vi "Data Log Refresh.vi"(8 "error in (no error)":errorcluster, 11 "Data Cluster":T1) -> (0 "error out":errorcluster)   [LabVIEW 2025]
uses:
  controls/LAB-IQ UI Data.ctl
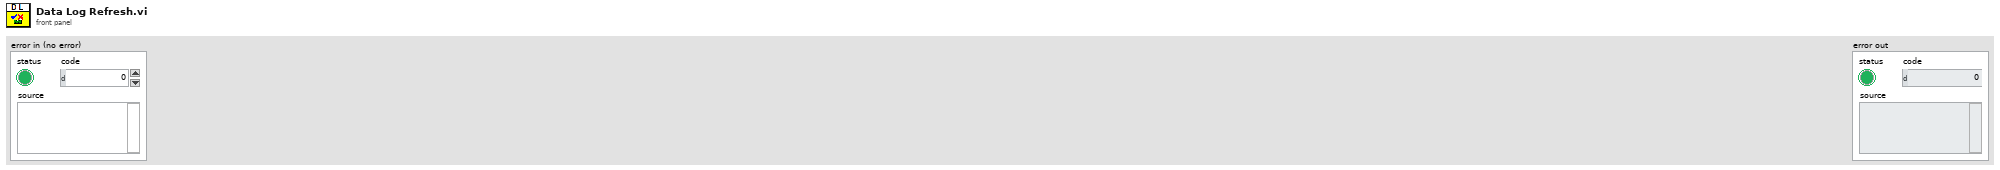
[diagram p1: front panel]
types:
  T1 = typedef "LAB-IQ UI Data.ctl" = cluster{"Main Home Screen":cluster{"GUI":refnum<vi>, "Platform Settings":refnum<vi>, "Configure":refnum<vi>, "Home":refnum<vi>, "EXIT":refnum<vi>, "service 2":refnum<vi>, "MainPage":refnum<vi>, "Analysis":refnum<vi>}, "Platform Settings":cluster{"mm/s  Surge":refnum<vi>, "Update Surge Speed":refnum<vi>, "Drive Error":refnum<vi>, "Disable Axis Jog Soft Limits":refnum<vi>, "mm/s  Sway":refnum<vi>, "Sway and Surge COM Status":refnum<vi>, "Heave COM Status":refnum<vi>, "Enable Platform":refnum<vi>, "Surge Forward Main":refnum<vi>, "Sway Right Main":refnum<vi>, "Sway Left Main":refnum<vi>, "Heave Down Main":refnum<vi>, "Heave Up main":refnum<vi>, "Update Sway Speed":refnum<vi>, "Update Heave Speed":refnum<vi>, "mm/s Heave":refnum<vi>, "mm/sec":refnum<vi>, "mm":refnum<vi>, "Surge Backward Main":refnum<vi>}, "Analysis Screen":cluster{"Analysis Home":refnum<vi>, "Surface Analysis":refnum<vi>, "Imaging":refnum<vi>, "Image Analysis":refnum<vi>, "Post Analysis":refnum<vi>}, "Config Screen":cluster{"Select Load Head":refnum<vi>, "Notes :":refnum<vi>, "FILE":refnum<vi>, "Sample ID :":refnum<vi>, "Operator ID :":refnum<vi>, "Operator Name :":refnum<vi>, "Auto":refnum<vi>}, "Motion Module":cluster{"zNL":refnum<vi>, "NL disp":refnum<vi>, "Rotary Tab":refnum<vi>, "Motion Direction:  3":refnum<vi>, "E.Velocity 2":refnum<vi>, "e.v/ssr 2":refnum<vi>, "Enter Fixed E.Velocity 2":refnum<vi>, "Enter Final SRR 2":refnum<vi>, "Enter initial SRR 2":refnum<vi>, "Enter Fixed SRR 2":refnum<vi>, "Enter the Final E.Velocity (m/s) 2":refnum<vi>, "Enter initial E.Velocity (m/s) 2":refnum<vi>, "Final Speed (RPM) 3":refnum<vi>, "Initial Speed (RPM) 2":refnum<vi>, "Enter the Final Velocity (m/s) 3":refnum<vi>, "Enter initial Velocity (m/s)  3":refnum<vi>, "Ramp Up 2":refnum<vi>, "TEST SELECTION":refnum<vi>, "SPEED SELECTION : ":refnum<vi>, "Angular Oscillation Set":refnum<vi>, "Traction":refnum<vi>, "Step Speed":refnum<vi>, "StepTable For Load-Speed":refnum<vi>, "StepTable For Speed":refnum<vi>, "Surge Forward MM":refnum<vi>, "Surge Backward MM":refnum<vi>, "M3 Image":refnum<vi>, "String 39":refnum<vi>, "Sway Left MM":refnum<vi>, "Sway Right MM":refnum<vi>, "Disable Axis Jog Soft Limits":refnum<vi>, "mm":refnum<vi>, "Heave Down MM":refnum<vi>, "Heave Up MM":refnum<vi>, "Wear Track Diameter (mm)":refnum<vi>, "Set WTD":refnum<vi>, "HomeScratch":refnum<vi>, "HomeRot":refnum<vi>, "PlaceModule":refnum<vi>, "Enter the Angle (Deg)":refnum<vi>, "Enter the Frequency (Hz)":refnum<vi>, "Motion Mode:":refnum<vi>, "LR Sway":refnum<vi>, "Rot Hor":refnum<vi>, "Scratch":refnum<vi>, "LR Cam":refnum<vi>, "MMBack":refnum<vi>, "MMNext":refnum<vi>, "Rot Ver":refnum<vi>, "Rotary Module Selection":refnum<vi>, "calculate rotary":refnum<vi>, "SPEED SELECTION : rotary":refnum<vi>, "Import 2":refnum<vi>, "Save 2":refnum<vi>, "File Path :  2":refnum<vi>, "String 45":refnum<vi>, "StepTable For Speed 3":refnum<vi>, "Enter the Speed(mm/sec)":refnum<vi>, "Enter the Speed(RPM)":refnum<vi>, "Enter Scratch Speed (mm/s):":refnum<vi>, "SwaySpeed Set":refnum<vi>, "Scartch Offset":refnum<vi>, "Motion type:":refnum<vi>, "HomeScratch 2":refnum<vi>, "Enter Scratch length (mm):":refnum<vi>, "Wear Track Diameter":refnum<vi>, "Rotary Speed Exced":refnum<vi>, "Scratch Mode":refnum<vi>, "No of Scratch":refnum<vi>}, "Environmental control":cluster{"Humidity  Status  3":refnum<vi>, "Low Temp  Status  2":refnum<vi>, "TK4 status 2":refnum<vi>, "Stage Temperature":refnum<vi>, "Sample Temperature":refnum<vi>, "Humidity (Amb)":refnum<vi>, "Clear List":refnum<vi>, "Add to list":refnum<vi>, "Wear":refnum<vi>, "Vibration":refnum<vi>, "Humidity (Chamber)":refnum<vi>, "Temperature (Chamber)":refnum<vi>, "ECR ":refnum<vi>, "Temperature (Amb)":refnum<vi>, "Microphone":refnum<vi>, "Acoustic Emission 3":refnum<vi>, "SNext":refnum<vi>, "APBack":refnum<vi>, "Enter the Temperature (°C):":refnum<vi>, "Enter the Stage \nTemperature (°C):":refnum<vi>, "Enter the Humidity (%Rh):":refnum<vi>, "Low Temp":refnum<vi>, "High Temp":refnum<vi>, "Humidity":refnum<vi>, "Sensors Picked":refnum<vi>}, "About Screen":cluster{"Password":refnum<vi>, "Home Service":refnum<vi>, "Advanced Setting":refnum<vi>, "About Tab":refnum<vi>, "ECR Port:":refnum<vi>, "Ramp Port:":refnum<vi>, "Installation/Replacement completed":refnum<vi>, "Loahead":refnum<vi>, "Heave and Surge COM Port:":refnum<vi>, "Sway COM Port:":refnum<vi>, "Temp Modbus:":refnum<vi>, "Humidity Port:":refnum<vi>, "Edit Gain Constants":refnum<vi>, "Save Gain Constants":refnum<vi>}, "Main Screen":cluster{"Main Screen Tab":refnum<vi>, "Angle and Frequency":refnum<vi>, "Stroke (mm)":refnum<vi>, "Angle (Deg)":refnum<vi>, "Main Speed Tab":refnum<vi>, "MTM MOTOR DISPLAY":refnum<vi>, "Disc Speed (m/sec)":refnum<vi>, "Ball Speed (m/sec)":refnum<vi>, "Disc Speed (RPM)":refnum<vi>, "Ball Speed (RPM)":refnum<vi>, "SPEED TAB":refnum<vi>, "Speed (m/sec)":refnum<vi>, "Set Speed (m/sec)":refnum<vi>, "Speed (RPM)":refnum<vi>, "Set Speed":refnum<vi>, "Time Tab":refnum<vi>, "Time ( HH:MM:SS ) 2":refnum<vi>, "Test Duration":refnum<vi>, "Test Duration 4":refnum<vi>, "TEST CYCLE":refnum<vi>, "TOTAL CYCLES":refnum<vi>, "Set Load (N)":refnum<vi>, "Temp Tabs":refnum<vi>, "Heater":refnum<vi>, "TK4 status":refnum<vi>, "ChamberTemp":refnum<vi>, "SetTmp":refnum<vi>, "Controller  Status":refnum<vi>, "ChamberTemp 2":refnum<vi>, "SetTmp 2":refnum<vi>, "Controller  Status 2":refnum<vi>, "ChamberTemp 3":refnum<vi>, "SetTmp 3":refnum<vi>, "Cooling":refnum<vi>, "Load Communication":refnum<vi>, "Ambient \nTemperature":refnum<vi>, "HumCOMStatus":refnum<vi>, "Ambient\n Humidity":refnum<vi>, "Freq (Hz)":refnum<vi>, "Load En":refnum<vi>, "NLt":refnum<vi>, "zNL 2":refnum<vi>, "Humidity On":refnum<vi>, "humidity disp":refnum<vi>, "Set Humidity":refnum<vi>, "NL disp 2":refnum<vi>, "Humidity On 2":refnum<vi>, "humidity disp 2":refnum<vi>, "Set Humidity 2":refnum<vi>, "NL disp 3":refnum<vi>, "AppLoadSeq scratch":refnum<vi>, "Stop Scratch":refnum<vi>, "ClrLog":refnum<vi>, "Trip Log":refnum<vi>, "STOP":refnum<vi>, "Start Test":refnum<vi>, "Test status":refnum<vi>, "AR Led":refnum<vi>, "Data":refnum<vi>, "Health":refnum<vi>, "Sway COM Status":refnum<vi>, "Heave COM Status":refnum<vi>, "Grp Tab":refnum<vi>, "Sub Graph":refnum<vi>, "SD (mm)":refnum<vi>, "Siliding distance Reset Graph":refnum<vi>, "SDGp":refnum<vi>, "Humidity Reset Graph":refnum<vi>, "HumrGp":refnum<vi>, "Acoustic Emission (mV)":refnum<vi>, "Aqucostic Reset Graph":refnum<vi>, "gACQUOS":refnum<vi>, "ECR RESET":refnum<vi>, "ECR":refnum<vi>, "Temperature Reset":refnum<vi>, "Acoustic Emission (mV) 2":refnum<vi>, "Aqucostic Reset Graph 2":refnum<vi>, "gACQUOS 2":refnum<vi>, "ECR RESET 2":refnum<vi>, "ECR 2":refnum<vi>, "Temperature Reset 2":refnum<vi>, "Temperature (deg c)":refnum<vi>, "Speed Reset Graph":refnum<vi>, "Speed Tab":refnum<vi>, "MTM DISC  SPEED":refnum<vi>, "MTM BALL SPEED":refnum<vi>, "speed mm/sec":refnum<vi>, "Hymidity":refnum<vi>, "Humidity Disable trip":refnum<vi>, "CoF Trip  2":refnum<vi>, "Depth Trip":refnum<vi>, "Weart Deapth":refnum<vi>, "Depth Reset Graph":refnum<vi>, "Weart":refnum<vi>, "Depthz":refnum<vi>, "Depth (µm)":refnum<vi>, "WearGp":refnum<vi>, "NL Trip 2":refnum<vi>, "Load pid":refnum<vi>, "Load Disable Trip":refnum<vi>, "Load Reset Graph":refnum<vi>, "NL Display 4":refnum<vi>, "Main Chart 3":refnum<vi>, "BACK":refnum<vi>, "Depth Trip 2":refnum<vi>, "COF TRIP ":refnum<vi>, "Friction Force (N)":refnum<vi>, "FF Reset Graph":refnum<vi>, "FF Disable Trip":refnum<vi>, "FF TRIP":refnum<vi>, "COF Disable Trip":refnum<vi>, "COF Reset Graph":refnum<vi>, "Start Test Temp":refnum<vi>, "zFF":refnum<vi>, "Friction Force (N) Graph":refnum<vi>, "Coefficient of Friction":refnum<vi>, "Scratch Start Test":refnum<vi>, "FF Tab":refnum<vi>, "Cyclic Friction Force (N)":refnum<vi>, "CZ FF":refnum<vi>, "Cyclic Friction Force (N) Graph":refnum<vi>, "Cyclic Coefficient of Friction":refnum<vi>, "Cyclic FF TRIP":refnum<vi>, "Cyclic FF Disable Trip":refnum<vi>, "cyclic COF Disable Trip":refnum<vi>, "cyclic COF TRIP":refnum<vi>, "cyclic COF Reset Graph":refnum<vi>, "Cyclic FF Reset Graph":refnum<vi>, "Test Trip":refnum<vi>, "Multi Scratch Pass":refnum<vi>, "Scratch Start Recording":refnum<vi>}, "Loading":cluster{"Indentation":refnum<vi>, "Reference Sample":refnum<vi>, "Load Cell Communication Slide":refnum<vi>, "com 3":refnum<vi>, "com":refnum<vi>, "DecaForce COM Status":refnum<vi>, "Update":refnum<vi>, "Clear 3":refnum<vi>, "seq":refnum<vi>, "Stribeck table":refnum<vi>, "Stribeck Table  For loading":refnum<vi>, "Loading Mode":refnum<vi>, "Enter the Final Load (N)":refnum<vi>, "Enter the CoF Trip":refnum<vi>, "Enter the Friction Force Trip":refnum<vi>, "Enter the Normal load Trip":refnum<vi>, "Enter the Load  (N)":refnum<vi>, "KiloForce":refnum<vi>, "DecaForce ":refnum<vi>, "MicroForce":refnum<vi>, "LHBack":refnum<vi>, "LHNext":refnum<vi>, "Enter the Loading Rate (N/min)":refnum<vi>, "Message":refnum<vi>, "Warning 2":refnum<vi>, "SSP 0.75":refnum<vi>, "SSP 0.5":refnum<vi>, "SSP 0.3":refnum<vi>, "Warning":refnum<vi>, "gui GIF":refnum<vi>, "Communication is established":refnum<vi>, "AppLoad 4":refnum<vi>, "Multipoint":refnum<vi>, "Load Selection":refnum<vi>}, "PID":cluster{"Ramp MulFac":refnum<vi>, "pulses LoadDiffRamp(2..10)":refnum<vi>, "PulseControlRamp(diff<=3N)":refnum<vi>, "SetLoadDeadband(%) Load(0-10N)":refnum<vi>, "PID gains out delay (microForce)":refnum<vi>, "Ramp":refnum<vi>, "Gain 2":refnum<vi>, "pulses LoadDiff(2..10)":refnum<vi>, "pulses LoadDiff(11..50)":refnum<vi>, "PulseControl(diff<=3N)":refnum<vi>, "SetLoadDeadband(%)  2":refnum<vi>, "Dummy Run":refnum<vi>, "Vertical load (N)":refnum<vi>, "AutoTune":refnum<vi>, "Offset 3 ":refnum<vi>, "apply load":refnum<vi>, "Offset  3":refnum<vi>, "apply load 2":refnum<vi>, "Enter ByPass Load":refnum<vi>, "reinit 3":refnum<vi>, "output range delay":refnum<vi>, "PID gains out delay":refnum<vi>, "Bypass Load":refnum<vi>, "pulsesSent":refnum<vi>, "pulses ":refnum<vi>, "actpid":refnum<vi>, "gFF Rot":refnum<vi>, "pulses LoadDiff(21..1000)":refnum<vi>, "Delay":refnum<vi>, "deadband":refnum<vi>}, "Config Parameters":cluster{"Tab Control 3":refnum<vi>, "Tab Control 19":refnum<vi>, "SAMPLES":refnum<vi>, "Re-initilaize":refnum<vi>, "Filter ON/OFF":refnum<vi>, "TracHomeSurgeOffsetCounts 10MM":refnum<vi>, "TracHomeSwayOffsetCounts 10MM":refnum<vi>, "Acoustic Emission:":refnum<vi>, "Apply Filter (FF)":refnum<vi>, "Filter% 2":refnum<vi>, "Apply Filter (Load)":refnum<vi>, "Filter% ":refnum<vi>, "Sway distance (mm)":refnum<vi>, "Surge distance (mm)":refnum<vi>, "DataSavingLoopDelay(ms)":refnum<vi>, "SAVE 2":refnum<vi>, "Enter Distance":refnum<vi>, "Sway Counts:":refnum<vi>, "Distance (mm): 3":refnum<vi>, "Surge Counts:":refnum<vi>, "Distance (mm): 2":refnum<vi>, "Distance (mm):":refnum<vi>, "Heave Counts:":refnum<vi>, "LRMHomeSurgeOffsetCounts":refnum<vi>, "LRMHomeSwayOffsetCounts":refnum<vi>, "TracHomeSurgeOffsetCounts 20MM":refnum<vi>, "TracHomeSwayOffsetCounts 20MM":refnum<vi>, "RotHomeSwayOffsetCounts":refnum<vi>, "RotHomeSurgeOffsetCounts":refnum<vi>, "Heave distance":refnum<vi>, "Zmm":refnum<vi>, "Heave Pulses/mm":refnum<vi>, "Surge Pulses/mm":refnum<vi>, "Sway Pulses/mm":refnum<vi>, "Heave Pitch":refnum<vi>, "Surge Pitch":refnum<vi>, "Sway Pitch":refnum<vi>, "Heave PPR":refnum<vi>, "Surge PPR":refnum<vi>, "Sway PPR":refnum<vi>, "Tab Control 5":refnum<vi>, "Tab Control 14":refnum<vi>, "Tab Control 26":refnum<vi>, "AE":refnum<vi>, "Heave Loop Delay":refnum<vi>, "Heave PID Speed":refnum<vi>, "Surge Jog Speed":refnum<vi>, "Heave Jog Speed":refnum<vi>, "Sway Loop Delay":refnum<vi>, "Sway PID Speed":refnum<vi>, "Sway Jog Speed":refnum<vi>, "DEPTH TRIP VALUE":refnum<vi>, "LOAD TRIP VALUE":refnum<vi>, "DEPTH TRIP   ENABLE":refnum<vi>, "LOAD TRIP  ENABLE":refnum<vi>, "CYCLIC FF TRIP VALUE":refnum<vi>, "FF TRIP VALUE":refnum<vi>, "CYCLIC CoF TRIP VALUE":refnum<vi>, "COF TRIP VALUE":refnum<vi>, "CYCLIC COF TRIP  ENABLE":refnum<vi>, "CYCLIC FF TRIP  ENABLE":refnum<vi>, "FF TRIP  ENABLE":refnum<vi>, "COF TRIP  ENABLE":refnum<vi>}, "Loading Com Port":cluster{"ClearAll":refnum<vi>, "Mz(Nm)":refnum<vi>, "My(Nm)":refnum<vi>, "Mx(Nm)":refnum<vi>, "Save Dwell":refnum<vi>, "Mx ":refnum<vi>, "My ":refnum<vi>, "Mz":refnum<vi>, "Fx(N)":refnum<vi>, "Fy(N)":refnum<vi>, "Fz(N)":refnum<vi>, "ZeroAll":refnum<vi>, "Acq Delay (ms)":refnum<vi>, "Burst Delay (ms)":refnum<vi>, "model":refnum<vi>, "SN":refnum<vi>, "FFx(N)":refnum<vi>, "Sensor IP":refnum<vi>, "Port":refnum<vi>, "FFy(N)":refnum<vi>, "Load(N)":refnum<vi>, "delete Handle":refnum<vi>, "Create Handle":refnum<vi>, "ft_data":refnum<vi>, "ft_range":refnum<vi>, "ft_data 2":refnum<vi>, "stop 6":refnum<vi>, "running_flag":refnum<vi>, "ft_udp_handle":refnum<vi>, "get-data-return":refnum<vi>, "get-range-return":refnum<vi>, "zero-return":refnum<vi>, "filter-return":refnum<vi>, "initial-return":refnum<vi>, "deleteHandle-result":refnum<vi>, "Load Cell Temp":refnum<vi>}, "Heave AND Surge":cluster{"SURGE POSE":refnum<vi>, "error out Read":refnum<vi>, "HEAVE POSE":refnum<vi>, "State":refnum<vi>, "Homed":refnum<vi>, "Sequence ID":refnum<vi>, "error out Write":refnum<vi>, "faultCode":refnum<vi>, "Ack ID":refnum<vi>, "SPEED":refnum<vi>, "Distance":refnum<vi>, "Mode Command":refnum<vi>, "Heave and Surge Read":refnum<vi>, "Read Heave Temp":refnum<vi>, "Spare 15":refnum<vi>, "Spare 14":refnum<vi>, "Spare 13":refnum<vi>, "Spare 12":refnum<vi>, "Spare 11":refnum<vi>, "Spare 10":refnum<vi>, "Spare 9":refnum<vi>, "Spare 8":refnum<vi>, "Spare 7":refnum<vi>, "Spare 6":refnum<vi>, "Spare 5":refnum<vi>, "Spare 4":refnum<vi>, "Spare 2":refnum<vi>, "Spare 1":refnum<vi>, "Node Id":refnum<vi>, "Spare 3":refnum<vi>, "SPARE 4":refnum<vi>, "SPARE 3":refnum<vi>, "SPARE 2":refnum<vi>, "SPARE 1":refnum<vi>, "fwMajor":refnum<vi>, "fwMinor":refnum<vi>, "Manual Write":refnum<vi>, "Heave and Surge Write":refnum<vi>}, "New PID LOGIC":cluster{"Fine Tune Zone":refnum<vi>, "PID SDelay":refnum<vi>, "Max_pos_limit":refnum<vi>, "Min_pos_limit":refnum<vi>, "i_limit":refnum<vi>, "pct_scale":refnum<vi>, "Deadband":refnum<vi>, "Kd":refnum<vi>, "Ki":refnum<vi>, "Kp":refnum<vi>, "Current Position":refnum<vi>, "Set Load":refnum<vi>, "Current Load":refnum<vi>, "Pulse delta":refnum<vi>, "Init Step":refnum<vi>, "Max Step Linit":refnum<vi>}, "SWAY ":cluster{"fwMajor":refnum<vi>, "Homed":refnum<vi>, "Rotary POSE":refnum<vi>, "State":refnum<vi>, "SWAY POSE":refnum<vi>, "Ack ID":refnum<vi>, "faultCode":refnum<vi>, "Node Id":refnum<vi>, "fwMinor":refnum<vi>, "Spare 6":refnum<vi>, "Spare 5":refnum<vi>, "Spare 4":refnum<vi>, "Spare 3":refnum<vi>, "Spare 2":refnum<vi>, "Spare 1":refnum<vi>, "Spare 7":refnum<vi>, "SPARE  5":refnum<vi>, "error out Write  SWAY ":refnum<vi>, "error out Read SWAY ":refnum<vi>, "Manual Write SWAY ":refnum<vi>, "SWAY WRITE":refnum<vi>, "SPARE  4":refnum<vi>, "SPARE  3":refnum<vi>, "SPARE 2":refnum<vi>, "SPARE 1":refnum<vi>, "Spare 15":refnum<vi>, "Spare 14":refnum<vi>, "Spare 13":refnum<vi>, "Spare 12":refnum<vi>, "Spare 11":refnum<vi>, "Spare 9":refnum<vi>, "Spare 8":refnum<vi>, "SPEED":refnum<vi>, "Distance":refnum<vi>, "Mode Command":refnum<vi>, "Sequence ID":refnum<vi>, "SWAY READ":refnum<vi>, "Spare 10":refnum<vi>, "Read SWAY Temp":refnum<vi>}, "Analysis Screen":cluster{"Analysis Home":refnum<vi>, "Refresh 2":refnum<vi>, "MEAN 4":refnum<vi>, "SD 4":refnum<vi>, "VARIANCE 4":refnum<vi>, "MEAN  3":refnum<vi>, "SD  3":refnum<vi>, "VARIANCE  3":refnum<vi>, "MEAN 2":refnum<vi>, "SD  2":refnum<vi>, "VARIANCE 2":refnum<vi>, "MEAN":refnum<vi>, "SD":refnum<vi>, "VARIANCE":refnum<vi>, "File 4 Discription":refnum<vi>, "OPEN 4":refnum<vi>, "File Name 4":refnum<vi>, "OPEN 3":refnum<vi>, "File 3 Discription":refnum<vi>, "File Name 3":refnum<vi>, "Y-AXIS":refnum<vi>, "X-AXIS":refnum<vi>, "XY Graph":refnum<vi>, "File Name 2":refnum<vi>, "File Name 1":refnum<vi>, "OPEN 2":refnum<vi>, "OPEN 1":refnum<vi>, "File 1 Discription ":refnum<vi>, "File 2 Discription":refnum<vi>, "Export":refnum<vi>, "File Format":refnum<vi>}}
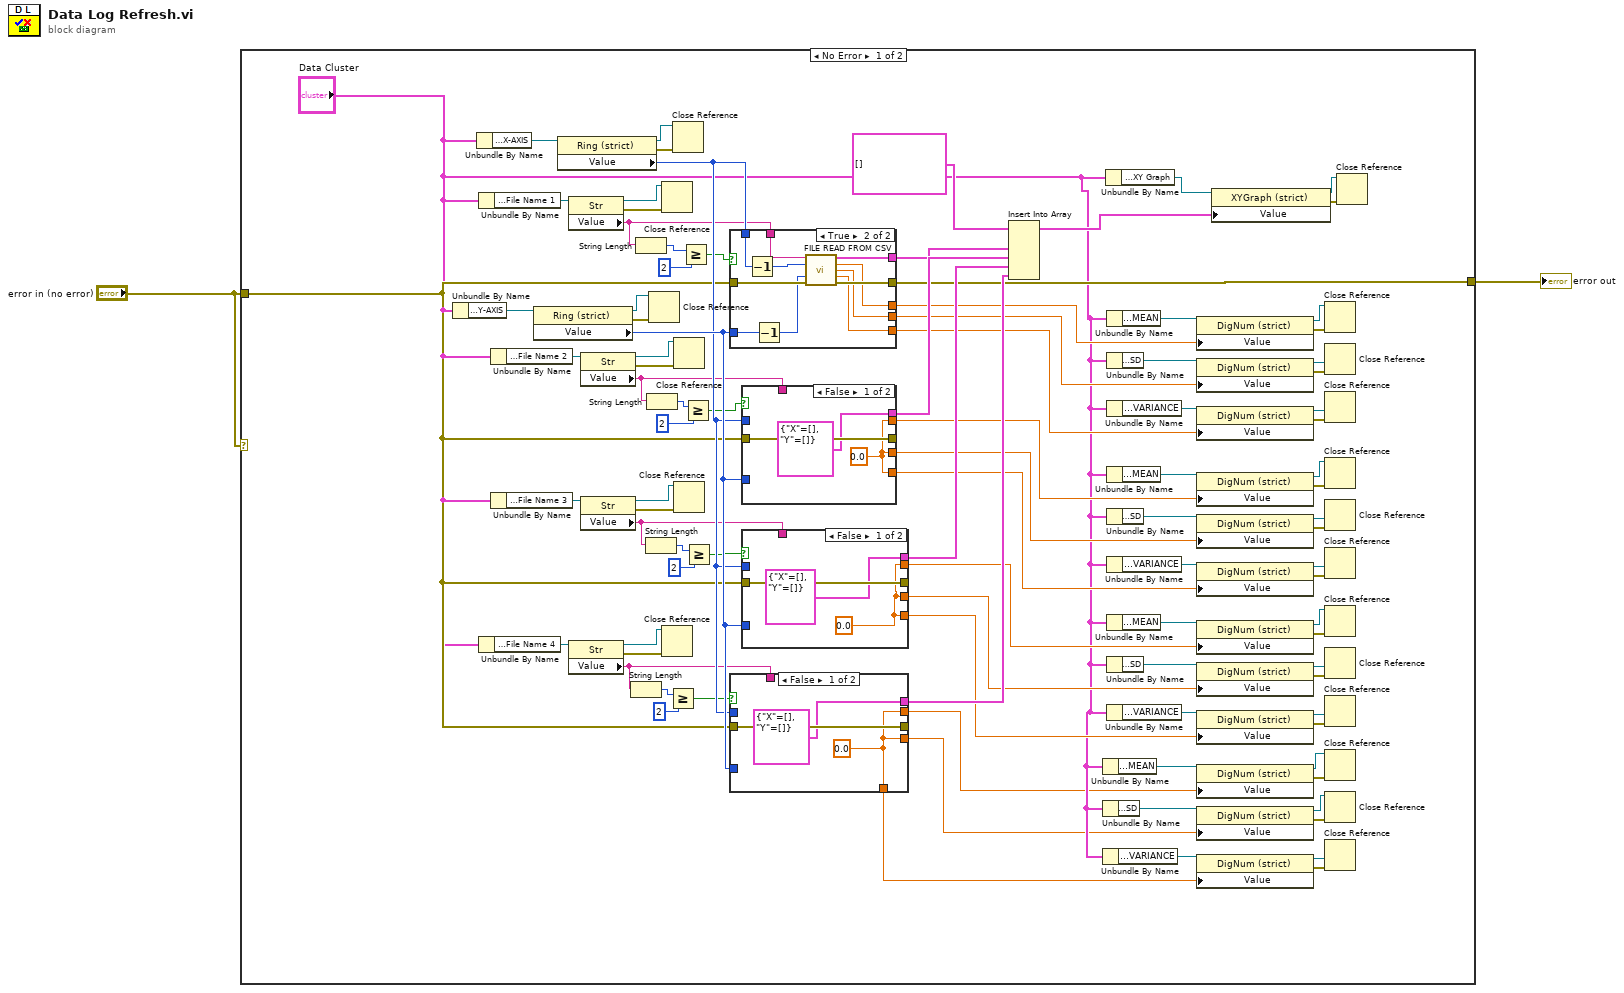
[diagram p0: block diagram]
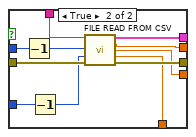
[diagram p2: hidden frame]
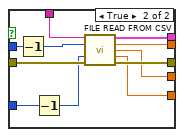
[diagram p3: hidden frame]
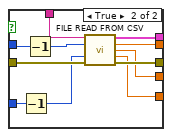
[diagram p4: hidden frame]
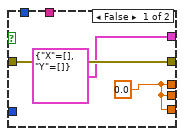
[diagram p5: hidden frame]
diagram:
  n1 = case shown="No Error" "error in (no error)" {
    tunnel: "error in (no error)" -> [w81 _]
    tunnel: [w55 _] -> w2
    frame No Error {
      n2 = Unbundle By Name("Data Cluster") -> ("Analysis Screen.Y-AXIS"=w94:refnum<vi>)
      n3 = Unbundle By Name("Data Cluster") -> ("Analysis Screen.X-AXIS"=w91:refnum<vi>)
      n4 = Unbundle By Name("Data Cluster") -> ("Analysis Screen.File Name 1"=w53:refnum<vi>)
      n5 = Unbundle By Name("Data Cluster") -> ("Analysis Screen.File Name 4"=w75:refnum<vi>)
      n6 = Unbundle By Name("Data Cluster") -> ("Analysis Screen.File Name 2"=w65:refnum<vi>)
      n7 = Unbundle By Name("Data Cluster") -> ("Analysis Screen.File Name 3"=w68:refnum<vi>)
      n8 = property class="Ring (strict)"(reference=w94) -> (reference out=w96:refnum<vi>, error out=w95:errorcluster, "Value"=w98:u16)  [unwired: 1 in]
      n9 = property class="Ring (strict)"(reference=w91) -> (reference out=w93:refnum<vi>, error out=w92:errorcluster, "Value"=w97:u16)  [unwired: 1 in]
      n10 = property class="Str"(reference=w53) -> (reference out=w52:refnum<vi>, error out=w54:errorcluster, "Value"=w56:string)  [unwired: 1 in]
      n11 = property class="Str"(reference=w75) -> (reference out=w74:refnum<vi>, error out=w76:errorcluster, "Value"=w77:string)  [unwired: 1 in]
      n12 = property class="Str"(reference=w65) -> (reference out=w66:refnum<vi>, error out=w64:errorcluster, "Value"=w63:string)  [unwired: 1 in]
      n13 = property class="Str"(reference=w68) -> (reference out=w67:refnum<vi>, error out=w69:errorcluster, "Value"=w70:string)  [unwired: 1 in]
      n14 = String Length(string=w77) -> (length=w78:i32)
      n15 = String Length(string=w56) -> (length=w57:i32)
      n16 = String Length(string=w70) -> (length=w71:i32)
      n17 = String Length(string=w63) -> (length=w62:i32)
      n18 = Close Reference(reference=w96, error in (no error)=w95) -> ()  [unwired: 1 out]
      n19 = Close Reference(reference=w52, error in (no error)=w54) -> ()  [unwired: 1 out]
      n20 = Close Reference(reference=w74, error in (no error)=w76) -> ()  [unwired: 1 out]
      n21 = Greater Or Equal?(x=w78, y=2) -> (x >= y?=w80:bool)
      n22 = Close Reference(reference=w93, error in (no error)=w92) -> ()  [unwired: 1 out]
      n23 = Close Reference(reference=w66, error in (no error)=w64) -> ()  [unwired: 1 out]
      n24 = Close Reference(reference=w67, error in (no error)=w69) -> ()  [unwired: 1 out]
      n25 = Greater Or Equal?(x=w57, y=2) -> (x >= y?=w59:bool)
      n26 = Greater Or Equal?(x=w62, y=2) -> (x >= y?=w60:bool)
      n27 = Greater Or Equal?(x=w71, y=2) -> (x >= y?=w73:bool)
      n28 = case shown="True" w59 {
        tunnel: w81 -> [w143 w154]
        tunnel: [w143 w153] -> w55
        tunnel: w56 -> [_ w152]
        tunnel: [cluster{"X":dbl[], "Y":dbl[]} {"X"=[], "Y"=[]} ("output cluster") w151] -> w86
        tunnel: w97 -> [_ w150]
        tunnel: w98 -> [_ w149]
        tunnel: [w141 w146] -> w42
        tunnel: [w141 w145] -> w41
        tunnel: [w141 w144] -> w40
        frame False {
          w141 = 0.0
        }
        frame True {
          n29 = Decrement(x=w150) -> (x-1=w148:u16)
          n30 = Decrement(x=w149) -> (x-1=w147:u16)
          n31 = call "FILE READ FROM CSV.vi"("File Path"=w152, "X-AXIS"=w148, "Y-AXIS"=w147, "error in (no error)"=w154) -> ("output cluster"=w151:cluster{"X":dbl[], "Y":dbl[]}, "mean"=w146:dbl, "standard deviation"=w145:dbl, "variance"=w144:dbl, "error out"=w153:errorcluster)  [unwired: 7 in]
        }
      }
      n32 = case shown="False" w80 {
        tunnel: w81 -> [w101 w112]
        tunnel: [w101 w111] -> _
        tunnel: w77 -> [_ w110]
        tunnel: [cluster{"X":dbl[], "Y":dbl[]} {"X"=[], "Y"=[]} ("output cluster") w109] -> w89
        tunnel: w97 -> [_ w108]
        tunnel: w98 -> [_ w106]
        tunnel: [w99 w104] -> w5
        tunnel: [w99 w103] -> w4
        tunnel: [w99 w102] -> w3
        frame False {
          w99 = 0.0
        }
        frame True {
          n33 = Decrement(x=w108) -> (x-1=w107:u16)
          n34 = Decrement(x=w106) -> (x-1=w105:u16)
          n35 = call "FILE READ FROM CSV.vi"("File Path"=w110, "X-AXIS"=w107, "Y-AXIS"=w105, "error in (no error)"=w112) -> ("output cluster"=w109:cluster{"X":dbl[], "Y":dbl[]}, "mean"=w104:dbl, "standard deviation"=w103:dbl, "variance"=w102:dbl, "error out"=w111:errorcluster)  [unwired: 7 in]
        }
      }
      n36 = case shown="False" w60 {
        tunnel: w81 -> [w129 w140]
        tunnel: [w129 w139] -> _
        tunnel: w63 -> [_ w138]
        tunnel: [cluster{"X":dbl[], "Y":dbl[]} {"X"=[], "Y"=[]} ("output cluster") w137] -> w87
        tunnel: w97 -> [_ w136]
        tunnel: w98 -> [_ w134]
        tunnel: [w127 w132] -> w30
        tunnel: [w127 w131] -> w29
        tunnel: [w127 w130] -> w28
        frame False {
          w127 = 0.0
        }
        frame True {
          n37 = Decrement(x=w134) -> (x-1=w133:u16)
          n38 = Decrement(x=w136) -> (x-1=w135:u16)
          n39 = call "FILE READ FROM CSV.vi"("File Path"=w138, "X-AXIS"=w135, "Y-AXIS"=w133, "error in (no error)"=w140) -> ("output cluster"=w137:cluster{"X":dbl[], "Y":dbl[]}, "mean"=w132:dbl, "standard deviation"=w131:dbl, "variance"=w130:dbl, "error out"=w139:errorcluster)  [unwired: 7 in]
        }
      }
      n40 = case shown="False" w73 {
        tunnel: w81 -> [w115 w126]
        tunnel: [w115 w125] -> _
        tunnel: w70 -> [_ w124]
        tunnel: [cluster{"X":dbl[], "Y":dbl[]} {"X"=[], "Y"=[]} ("output cluster") w123] -> w88
        tunnel: w97 -> [_ w122]
        tunnel: w98 -> [_ w120]
        tunnel: [w113 w118] -> w18
        tunnel: [w113 w117] -> w17
        tunnel: [w113 w116] -> w16
        frame False {
          w113 = 0.0
        }
        frame True {
          n41 = Decrement(x=w122) -> (x-1=w121:u16)
          n42 = Decrement(x=w120) -> (x-1=w119:u16)
          n43 = call "FILE READ FROM CSV.vi"("File Path"=w124, "X-AXIS"=w121, "Y-AXIS"=w119, "error in (no error)"=w126) -> ("output cluster"=w123:cluster{"X":dbl[], "Y":dbl[]}, "mean"=w118:dbl, "standard deviation"=w117:dbl, "variance"=w116:dbl, "error out"=w125:errorcluster)  [unwired: 7 in]
        }
      }
      n44 = Insert Into Array(array=cluster{"Array 2":dbl[], "Array 2":dbl[]}[] [] ("Value"), new element #1=w86, new element #2=w87, new element #3=w88, new element #4=w89) -> (w90:cluster{"Array 2":dbl[], "Array 2":dbl[]}[])  [unwired: 1 in]
      n45 = Unbundle By Name("Data Cluster") -> ("Analysis Screen.MEAN"=w8:refnum<vi>)
      n46 = Unbundle By Name("Data Cluster") -> ("Analysis Screen.SD"=w11:refnum<vi>)
      n47 = Unbundle By Name("Data Cluster") -> ("Analysis Screen.VARIANCE"=w14:refnum<vi>)
      n48 = Unbundle By Name("Data Cluster") -> ("Analysis Screen.XY Graph"=w83:refnum<vi>)
      n49 = Unbundle By Name("Data Cluster") -> ("Analysis Screen.MEAN"=w50:refnum<vi>)
      n50 = Unbundle By Name("Data Cluster") -> ("Analysis Screen.SD"=w47:refnum<vi>)
      n51 = Unbundle By Name("Data Cluster") -> ("Analysis Screen.VARIANCE"=w44:refnum<vi>)
      n52 = Unbundle By Name("Data Cluster") -> ("Analysis Screen.MEAN"=w32:refnum<vi>)
      n53 = Unbundle By Name("Data Cluster") -> ("Analysis Screen.SD"=w35:refnum<vi>)
      n54 = Unbundle By Name("Data Cluster") -> ("Analysis Screen.VARIANCE"=w38:refnum<vi>)
      n55 = Unbundle By Name("Data Cluster") -> ("Analysis Screen.MEAN"=w26:refnum<vi>)
      n56 = Unbundle By Name("Data Cluster") -> ("Analysis Screen.SD"=w23:refnum<vi>)
      n57 = Unbundle By Name("Data Cluster") -> ("Analysis Screen.VARIANCE"=w20:refnum<vi>)
      n58 = property class="DigNum (strict)"(reference=w50, "Value"=w42) -> (reference out=w49:refnum<vi>, error out=w51:errorcluster)  [unwired: 1 in]
      n59 = property class="DigNum (strict)"(reference=w47, "Value"=w41) -> (reference out=w48:refnum<vi>, error out=w46:errorcluster)  [unwired: 1 in]
      n60 = property class="DigNum (strict)"(reference=w44, "Value"=w40) -> (reference out=w43:refnum<vi>, error out=w45:errorcluster)  [unwired: 1 in]
      n61 = property class="DigNum (strict)"(reference=w32, "Value"=w30) -> (reference out=w33:refnum<vi>, error out=w31:errorcluster)  [unwired: 1 in]
      n62 = property class="DigNum (strict)"(reference=w35, "Value"=w29) -> (reference out=w34:refnum<vi>, error out=w36:errorcluster)  [unwired: 1 in]
      n63 = property class="DigNum (strict)"(reference=w38, "Value"=w28) -> (reference out=w39:refnum<vi>, error out=w37:errorcluster)  [unwired: 1 in]
      n64 = property class="DigNum (strict)"(reference=w26, "Value"=w18) -> (reference out=w25:refnum<vi>, error out=w27:errorcluster)  [unwired: 1 in]
      n65 = property class="DigNum (strict)"(reference=w23, "Value"=w17) -> (reference out=w24:refnum<vi>, error out=w22:errorcluster)  [unwired: 1 in]
      n66 = property class="DigNum (strict)"(reference=w20, "Value"=w16) -> (reference out=w19:refnum<vi>, error out=w21:errorcluster)  [unwired: 1 in]
      n67 = property class="DigNum (strict)"(reference=w8, "Value"=w5) -> (reference out=w9:refnum<vi>, error out=w7:errorcluster)  [unwired: 1 in]
      n68 = property class="DigNum (strict)"(reference=w11, "Value"=w4) -> (reference out=w10:refnum<vi>, error out=w12:errorcluster)  [unwired: 1 in]
      n69 = property class="DigNum (strict)"(reference=w14, "Value"=w3) -> (reference out=w15:refnum<vi>, error out=w13:errorcluster)  [unwired: 1 in]
      n70 = property class="XYGraph (strict)"(reference=w83, "Value"=w90) -> (reference out=w82:refnum<vi>, error out=w84:errorcluster)  [unwired: 1 in]
      n71 = Close Reference(reference=w49, error in (no error)=w51) -> ()  [unwired: 1 out]
      n72 = Close Reference(reference=w48, error in (no error)=w46) -> ()  [unwired: 1 out]
      n73 = Close Reference(reference=w43, error in (no error)=w45) -> ()  [unwired: 1 out]
      n74 = Close Reference(reference=w33, error in (no error)=w31) -> ()  [unwired: 1 out]
      n75 = Close Reference(reference=w34, error in (no error)=w36) -> ()  [unwired: 1 out]
      n76 = Close Reference(reference=w39, error in (no error)=w37) -> ()  [unwired: 1 out]
      n77 = Close Reference(reference=w25, error in (no error)=w27) -> ()  [unwired: 1 out]
      n78 = Close Reference(reference=w24, error in (no error)=w22) -> ()  [unwired: 1 out]
      n79 = Close Reference(reference=w19, error in (no error)=w21) -> ()  [unwired: 1 out]
      n80 = Close Reference(reference=w9, error in (no error)=w7) -> ()  [unwired: 1 out]
      n81 = Close Reference(reference=w10, error in (no error)=w12) -> ()  [unwired: 1 out]
      n82 = Close Reference(reference=w15, error in (no error)=w13) -> ()  [unwired: 1 out]
      n83 = Close Reference(reference=w82, error in (no error)=w84) -> ()  [unwired: 1 out]
    }
    frame Error {
    }
  }
  "error out" <- w2
